vi "第4題.vi"() -> ()   [LabVIEW 2017]
uses:
  <vilib>/Utility/file.llb/Read Delimited Spreadsheet (DBL).vi
  <vilib>/Analysis/NI_AALPro.lvlib
  <vilib>/gmath/NI_Gmath.lvlib
panel:
  out "相關係數":dbl format="%.7g"
  out "父母年紀與零用錢斜率":dbl
  out "總比例":dbl
  out "父方年紀大於母方家庭數":dbl
  out "all rows":dbl[][](array[numeric])
  in  "file path (dialog if empty)":path
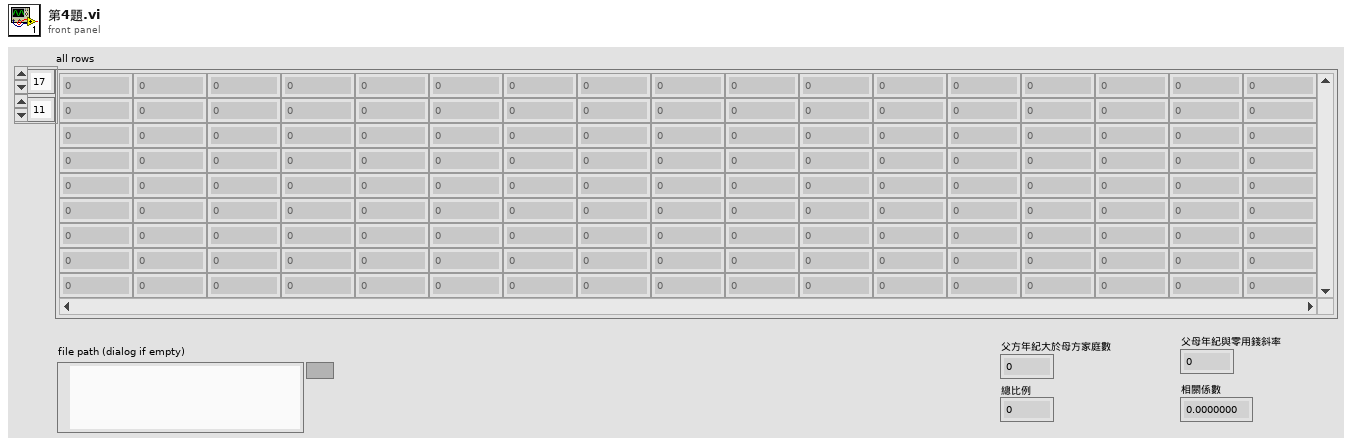
[diagram p1: front panel]
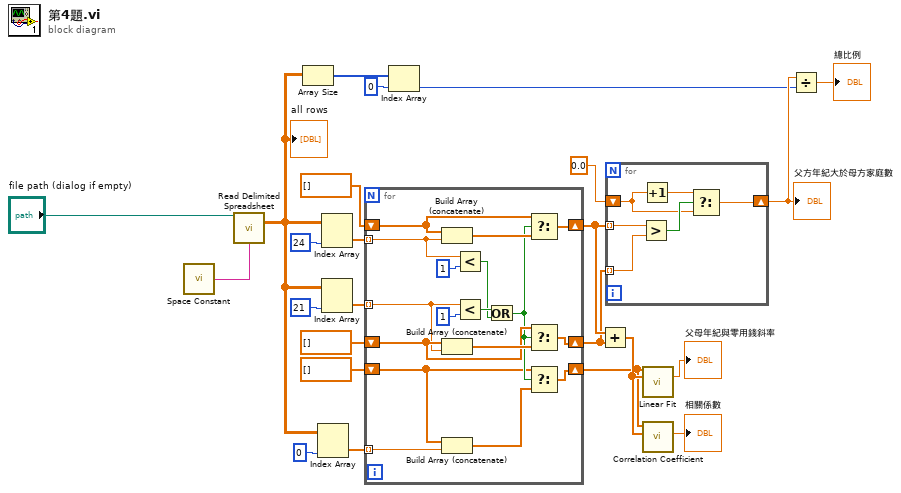
[diagram p0: block diagram]
diagram:
  n1 = call <vilib>:"Space Constant.vi"() -> ("String"=w23:string)
  n2 = call-poly <vilib>:"Read Delimited Spreadsheet.vi"("file path (dialog if empty)"="file path (dialog if empty)", "delimiter (\\t)"=w23) -> ("all rows"=w19:dbl[][])  [unwired: 8 in, 5 out]
  "all rows" <- w19
  n3 = Array Size(array=w19) -> (size(s)=w18:i32[])
  n4 = Index Array(array=w19, index (col)=0) -> (element=w6:dbl[])  [unwired: 1 in]
  n5 = Index Array(array=w19, index (col)=24) -> (element=w12:dbl[])  [unwired: 1 in]
  n6 = Index Array(array=w19, index (col)=21) -> (element=w13:dbl[])  [unwired: 1 in]
  n7 = for {
    tunnel: w13 -> [w32] mode=indexing
    tunnel: w12 -> [w30] mode=indexing
    shift-right: [w37] -> w7
    shift-left: dbl[] [] -> [w33]
    shift-right: [w34] -> w8
    shift-left: dbl[] [] -> [w31]
    tunnel: w6 -> [w25] mode=indexing
    shift-right: [w27] -> w2
    shift-left: dbl[] [] -> [w26]
    n8 = Build Array (concatenate)(w31, w30) -> (w35:dbl[])
    n9 = Build Array (concatenate)(w33, w32) -> (w36:dbl[])
    n10 = Build Array (concatenate)(w26, w25) -> (w29:dbl[])
    n11 = Less?(x=w30, y=1) -> (x < y?=w38:bool)
    n12 = Less?(x=w32, y=1) -> (x < y?=w39:bool)
    n13 = Or(x=w39, y=w38) -> (x .or. y?=w28:bool)
    n14 = Select(t=w31, s=w28, f=w35) -> (s? t:f=w34:dbl[])
    n15 = Select(t=w33, s=w28, f=w36) -> (s? t:f=w37:dbl[])
    n16 = Select(t=w26, s=w28, f=w29) -> (s? t:f=w27:dbl[])
  }
  n17 = Index Array(array=w18, index=0) -> (element=w15:i32)
  n18 = Add(x=w8, y=w7) -> (x+y=w3:dbl[])
  n19 = for {
    tunnel: w8 -> [w47] mode=indexing
    tunnel: w7 -> [w46] mode=indexing
    shift-right: [w44] -> w16
    shift-left: 0.0 -> [w43]
    n20 = Greater?(x=w47, y=w46) -> (0:w45:bool)
    n21 = Increment(x=w43) -> (x+1=w42:dbl)
    n22 = Select(t=w42, s=w45, f=w43) -> (s? t:f=w44:dbl)
  }
  "父方年紀大於母方家庭數" <- w16
  n23 = call <vilib>:"Linear Fit.vi"("Y"=w2, "X"=w3) -> ("slope"=→"父母年紀與零用錢斜率":dbl)  [unwired: 9 in, 4 out]
  n24 = call <vilib>:"Correlation Coefficient.vi"("Y"=w3, "X"=w2) -> ("r^2"=→"相關係數":dbl)  [unwired: 8 in, 1 out]
  n25 = Divide(x=w16, y=w15) -> (x/y=→"總比例":dbl)
